vi "build XY graph.vi"(0 "Gcode line":string, 2 "XY Graph in":cluster{"X":dbl, "Y":dbl}[](array[cluster])) -> (6 "XY Graph out":cluster{"X":dbl, "Y":dbl}[](array[cluster]))   [LabVIEW 2020]
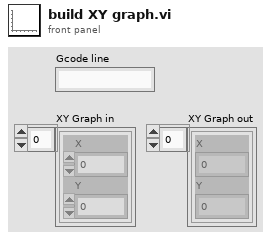
[diagram p1: front panel]
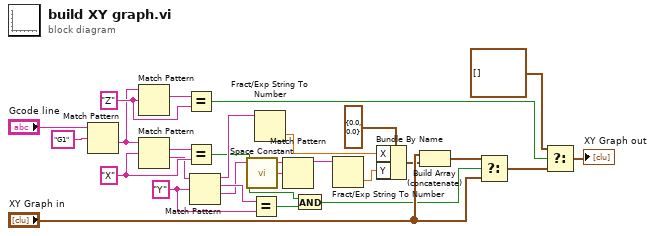
[diagram p0: block diagram]
diagram:
  w18 = "Z" ("regular expression")
  w8 = "Y" ("regular expression")
  w6 = "X" ("regular expression")
  n1 = Match Pattern(string="Gcode line", regular expression="G1") -> (after substring=w16:string)  [unwired: 1 in, 3 out]
  n2 = Match Pattern(string=w16, regular expression=w18) -> (match substring=w17:string)  [unwired: 1 in, 3 out]
  n3 = Match Pattern(string=w16, regular expression=w6) -> (match substring=w5:string, after substring=w2:string)  [unwired: 1 in, 2 out]
  n4 = Equal?(x=w17, y=w18) -> (x = y?=w24:bool)
  n5 = Equal?(x=w5, y=w6) -> (x = y?=w9:bool)
  n6 = Match Pattern(string=w2, regular expression=w8) -> (before substring=w11:string, match substring=w7:string, after substring=w3:string)  [unwired: 1 in, 1 out]
  n7 = call <vilib>:"Space Constant.vi"() -> ("String"=w4:string)
  n8 = Equal?(x=w7, y=w8) -> (x = y?=w10:bool)
  n9 = Fract/Exp String To Number(string=w11) -> (number=w14:dbl)  [unwired: 3 in, 1 out]
  n10 = Match Pattern(string=w3, regular expression=w4) -> (before substring=w12:string)  [unwired: 1 in, 3 out]
  n11 = And(x=w9, y=w10) -> (x .and. y?=w19:bool)
  n12 = Fract/Exp String To Number(string=w12) -> (number=w15:dbl)  [unwired: 3 in, 1 out]
  n13 = Bundle By Name(cluster=cluster{"X":dbl, "Y":dbl} {"X"=0.0, "Y"=0.0} ("XY Graph"), "X"=w14, "Y"=w15) -> (w21:cluster{"X":dbl, "Y":dbl})
  n14 = Build Array (concatenate)("XY Graph in", w21) -> (w20:cluster{"X":dbl, "Y":dbl}[])
  n15 = Select(t=w20, s=w19, f="XY Graph in") -> (s? t:f=w25:cluster{"X":dbl, "Y":dbl}[])
  n16 = Select(t=cluster{"X":dbl, "Y":dbl}[] [], s=w24, f=w25) -> (s? t:f=→"XY Graph out":cluster{"X":dbl, "Y":dbl}[])
